vi "Parse GLL.vi"(8 "error in (no error)":errorcluster, 10 "Message":refnum<class "NMEA Message.lvclass">, 11 "nmea in":refnum<class "nmea.lvclass">) -> (0 "error out":errorcluster, 3 "nmea out":refnum<class "nmea.lvclass">)   [LabVIEW 2020, in "nmea.lvlib" / "nmea.lvclass"]
uses:
  nmea.lvclass
  message/NMEA Message.lvclass
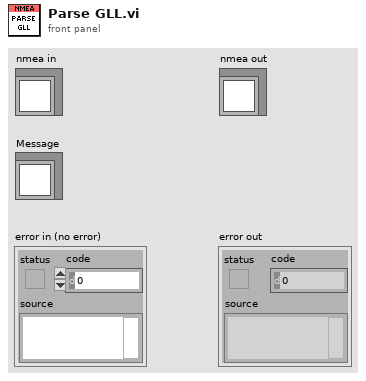
[diagram p1: front panel]
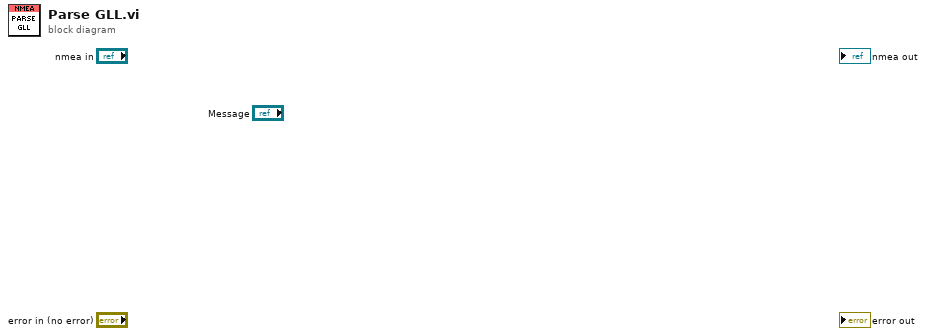
[diagram p0: block diagram]
diagram:
